vi "Send Handle Last Ack.vi"(9 "Error Report":errorcluster, 10 "State":variant, 11 "Ident":string) -> (2 "Message Out":T1)   [LabVIEW 2025]
uses:
  <extravilib>/ChannelInstances/Event Messenger-c(str,var)/))Channel.ctl
  Last Ack.ctl
  <extravilib>/ChannelInstances/Event Messenger-c(str,var)/))Channel.vi
  <extravilib>/ChannelInstances/Event Messenger-c(str,var).lvlib
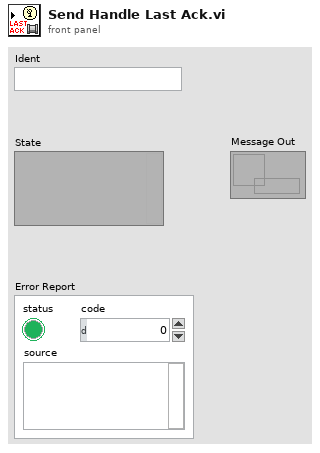
[diagram p1: front panel]
types:
  T1 = typedef "Event Messenger-c(str,var).lvlib/))Channel.ctl" = refnum<queue>
  T2 = typedef "Last Ack.ctl" = cluster{"Ident":string, "Error Report":errorcluster, "State ":string}
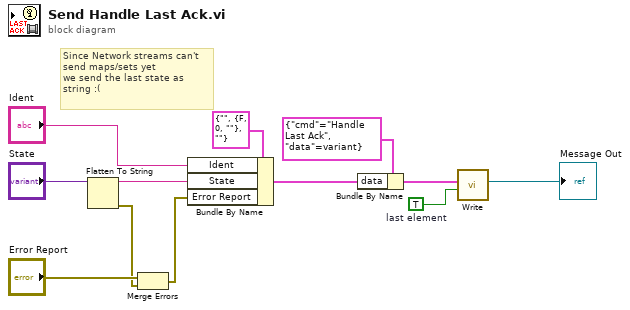
[diagram p0: block diagram]
diagram:
  w6 = TRUE  # last element
  # "Since Network streams can't\nsend maps/sets yet\nwe send the last state as\nstring :("
  n1 = Flatten To String(anything="State") -> (data string=w3:string, error out=w1:errorcluster)  [unwired: 3 in, 1 out]
  n2 = Merge Errors("Error Report", w1) -> (w2:errorcluster)
  n3 = Bundle By Name(cluster=T2 {"Ident"="", "Error Report"={"status"=FALSE, "code"=0, "source"=""}, "State "=""} ("Last Ack"), "Ident"="Ident", "State"=w3, "Error Report"=w2) -> (w12:T2)
  n4 = Bundle By Name(cluster=cluster{"cmd":string, "data":variant} {"cmd"="Handle Last Ack", "data"=variant} ("message"), "data"=w12) -> (w7:cluster{"cmd":string, "data":variant})
  n5 = call <extravilib>:"Write.vi"("last element? (F)"=w6, "element"=w7) -> ("channel"=→"Message Out":T1)  [unwired: 8 in, 1 out]
